vi "open connection.vi"(8 "error in (no error)":errorcluster, 11 "tcp server connection in":refnum<class "tcp server connection.lvclass">) -> (0 "error out":errorcluster, 3 "tcp server connection out":refnum<class "tcp server connection.lvclass">)   [LabVIEW 2014, in "tcp server connection.lvclass"]
uses:
  tcp server connection.lvclass
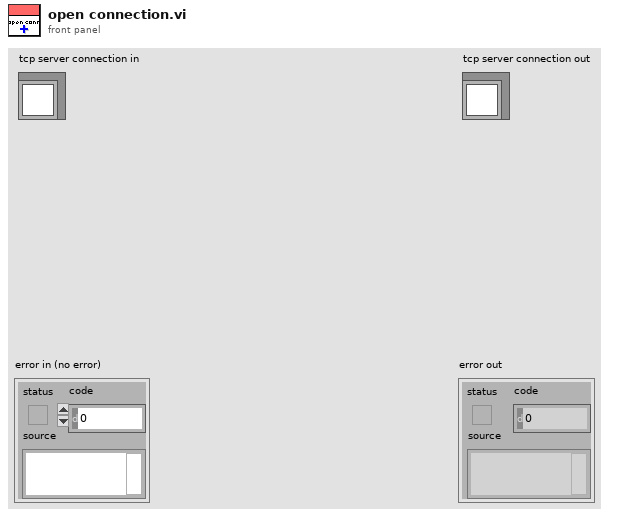
[diagram p1: front panel]
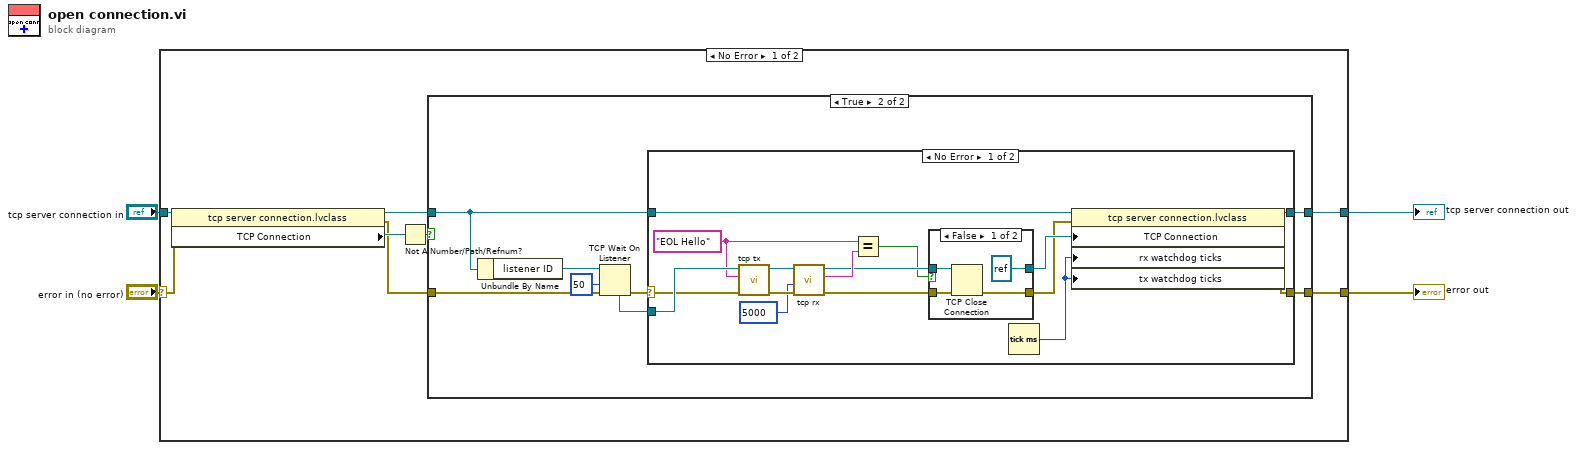
[diagram p0: block diagram]
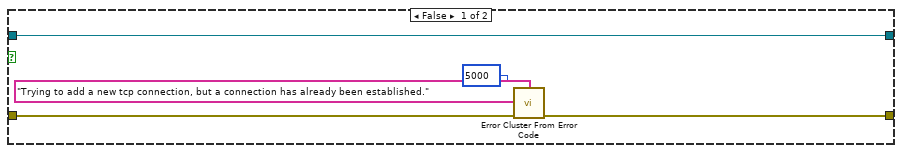
[diagram p2: hidden frame]
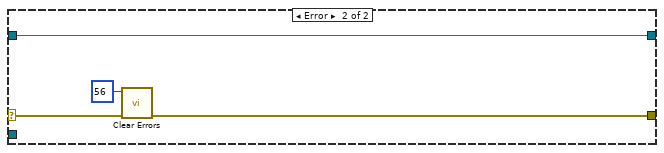
[diagram p4: hidden frame]
diagram:
  n1 = case shown="No Error" "error in (no error)" {
    selector: "error in (no error)" -> [w6 w53]
    tunnel: [w11 w53] -> w3
    tunnel: [w12 w52] -> w1
    tunnel: "tcp server connection in" -> [w9 w52]
    frame No Error {
      n2 = property class="tcp server connection.lvclass"(reference=w9, error in=w6) -> (reference out=w8:refnum<class "tcp server connection.lvclass">, error out=w5:errorcluster, "TCP Connection"=w7:refnum<k5>)
      n3 = Not A Number/Path/Refnum?(number/path/refnum=w7) -> (NaN/Path/Refnum?=w10:bool)
      n4 = case shown="True" w10 {
        tunnel: [w13 w25] -> w12
        tunnel: [w14 w24] -> w11
        tunnel: w5 -> [w15 w19]
        tunnel: w8 -> [w13 w18]
        frame False {
          n5 = call <vilib>:"Error Cluster From Error Code.vi"("error in (no error)"=w15, "error message (\"\")"="Trying to add a new tcp connection, but a connection has already been established." ("error message (\"\")"), "error code (0)"=5000) -> ("error out"=w14:errorcluster)  [unwired: 6 in]
        }
        frame True {
          n6 = Unbundle By Name(w18) -> ("listener ID"=w23:refnum<k5>)
          n7 = TCP Wait On Listener(8:w19, 9:50 ("timeout ms (wait forever: -1)"), 11:w23) -> (0:w21:errorcluster, 4:w20:refnum<k5>)  [unwired: 1 in, 3 out]
          n8 = case shown="No Error" w21 {
            selector: w21 -> [w32 w50]
            tunnel: w20 -> [w41 _]
            tunnel: [w30 w48] -> w25
            tunnel: [w27 w49] -> w24
            tunnel: w18 -> [w31 w48]
            frame No Error {
              w38 = "EOL Hello" ("data in")
              n9 = call "tcp tx.vi"("error in"=w32, "tx"=w38, "TCP Connection in"=w41) -> ("error out"=w39:errorcluster, "TCP Connection out"=w40:refnum<k5>)  [unwired: 7 in]
              n10 = call "tcp rx.vi"("error in"=w39, "poll timeout ms (50)"=5000 ("timeout ms (25000)"), "TCP Connection in"=w40) -> ("error out"=w34:errorcluster, "rx"=w37:string, "TCP Connection out"=w35:refnum<k5>)  [unwired: 5 in, 1 out]
              n11 = Equal?(x=w38, y=w37) -> (x = y?=w33:bool)
              n12 = case shown="False" w33 {
                tunnel: [refnum<k5> refnum ("TCP Connection out") w47] -> w29
                tunnel: w35 -> [w44 w47]
                tunnel: w34 -> [w45 w46]
                tunnel: [w43 w46] -> w28
                frame False {
                  n13 = TCP Close Connection(connection ID=w44, error in (no error)=w45) -> (error out=w43:errorcluster)  [unwired: 1 in, 1 out]
                }
                frame True {
                }
              }
              n14 = Tick Count (ms)() -> (millisecond timer value=w26:u32)
              n15 = property class="tcp server connection.lvclass"(reference=w31, error in=w28, "TCP Connection"=w29, "rx watchdog ticks"=w26, "tx watchdog ticks"=w26) -> (reference out=w30:refnum<class "tcp server connection.lvclass">, error out=w27:errorcluster)
            }
            frame Error {
              n16 = call <vilib>:"Clear Errors.vi"("error in (no error)"=w50, "specific error code to clear (0: all)"=56) -> ("error out"=w49:errorcluster)  [unwired: 4 in, 1 out]
            }
          }
        }
      }
    }
    frame Error {
    }
  }
  "error out" <- w3
  "tcp server connection out" <- w1
